vi "Producto select Process.vi"(8 "error in (no error)":errorcluster, 10 "Seleccionar Producto":enum16{"Coca", "Fanta", "Manzanita", "Ciel"}(ring), 11 "Soda Actor in":refnum<class "Soda Actor.lvclass">) -> (0 "error out":errorcluster, 3 "Soda Actor out":refnum<class "Soda Actor.lvclass">)   [LabVIEW 2020, in "Soda Actor.lvlib" / "Soda Actor.lvclass"]
uses:
  Soda Actor.lvclass
  Soda Actor.lvclass/Soda Actor.ctl
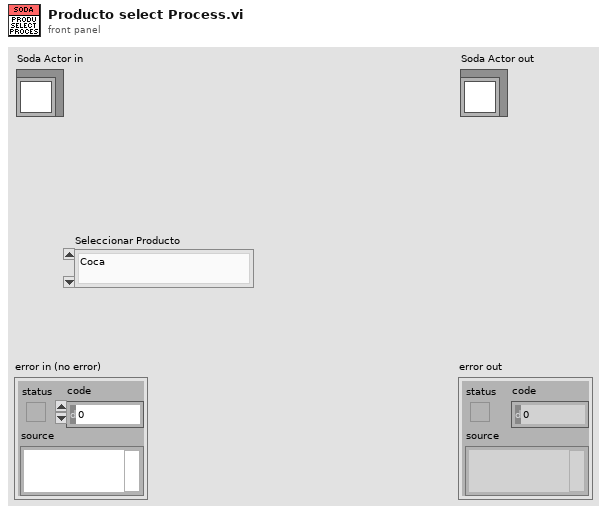
[diagram p1: front panel]
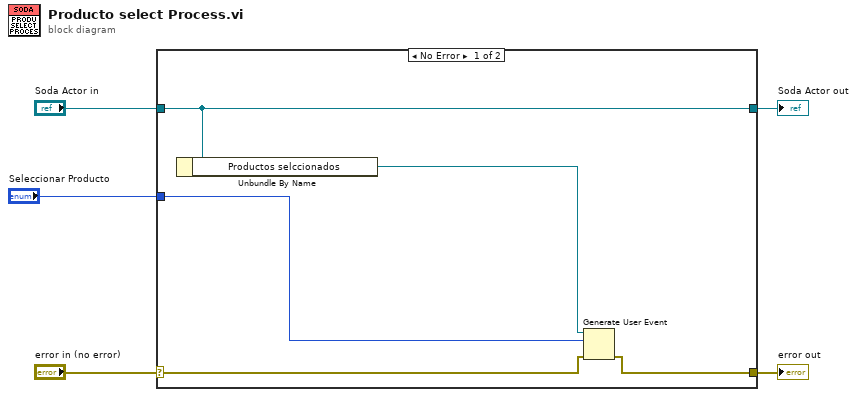
[diagram p0: block diagram]
diagram:
  n1 = case shown="No Error" "error in (no error)" {
    selector: "error in (no error)" -> [w8 w12]
    tunnel: [w9 w12] -> w4
    tunnel: [w10 w11] -> w2
    tunnel: "Soda Actor in" -> [w10 w11]
    tunnel: "Seleccionar Producto" -> [w6 _]
    frame No Error {
      n2 = Unbundle By Name(w10) -> ("Productos selccionados"=w7:refnum<user-event>)
      n3 = Generate User Event(user event=w7, event data cluster=w6, error in=w8) -> (error out=w9:errorcluster)  [unwired: 1 in, 1 out]
    }
    frame Error {
    }
  }
  "error out" <- w4
  "Soda Actor out" <- w2
